vi "globalSetUp.vi"(8 "error in (no error)":errorcluster, 11 "Instrument Addon Error System Tests in":refnum<class "Instrument Addon Error System Tests.lvclass">) -> (0 "error out":errorcluster, 3 "Instrument Addon Error System Tests out":refnum<class "Instrument Addon Error System Tests.lvclass">)   [LabVIEW 2019, in "Instrument Addon Error System Tests.lvclass"]
uses:
  Instrument Addon Error System Tests.lvclass
  C:/Program Files (x86)/National Instruments/LabVIEW 2019/vi.lib/NI/VeriStand Custom Device Testing Tools/VeriStandTestCase/VeriStandTestCase.lvclass
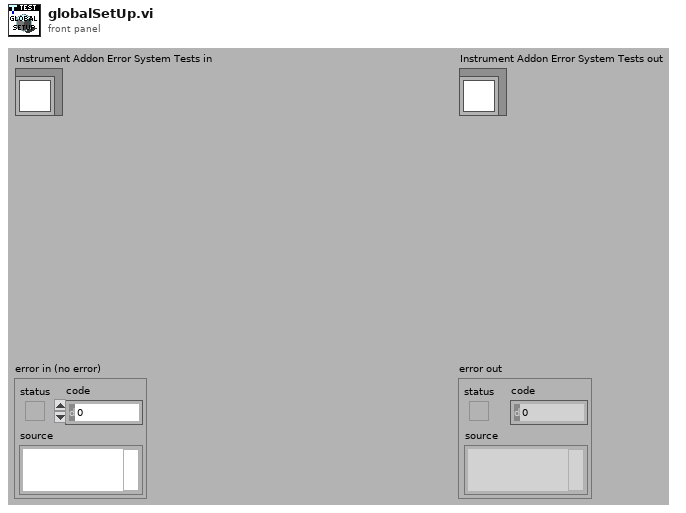
[diagram p1: front panel]
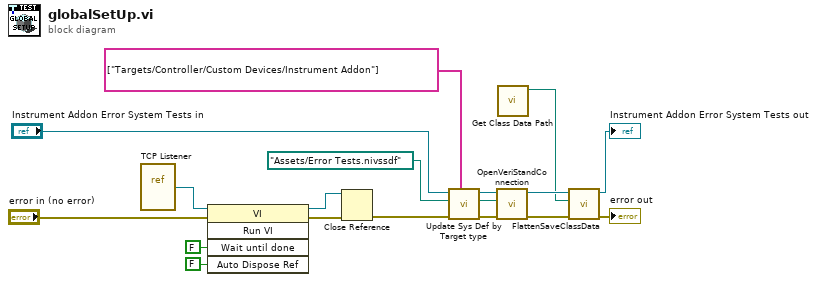
[diagram p0: block diagram]
diagram:
  n1 = vi-ref "TCP Listener.vi"() -> (w16:refnum<vi>)
  n2 = invoke class="VI" method="Run VI"(reference=w16, error in="error in (no error)", "Wait until done"=FALSE ("Wait Until Done"), "Auto Dispose Ref"=FALSE ("Auto Dispose Reference")) -> (reference out=w15:refnum<vi>, error out=w14:errorcluster)  [unwired: 1 in, 3 out]
  n3 = Close Reference(reference=w15, error in (no error)=w14) -> (error out=w5:errorcluster)
  n4 = call "Update Sys Def by Target type.vi"("nodepaths"=string[] ["Targets/Controller/Custom Devices/Instrument Addon"], "error in (no error)"=w5, "Sys Def relative path"=path "Assets/Error Tests.nivssdf" ("System Definition File"), "VeriStandTestCase in"="Instrument Addon Error System Tests in") -> ("error out"=w2:errorcluster, "Sys Def relative path out"=w3:path, "VeriStandTestCase out"=w6:refnum<class "Instrument Addon Error System Tests.lvclass">)  [unwired: 5 in]
  n5 = call-dynamic "OpenVeriStandConnection.vi"("error in (no error)"=w2, "System Definition File"=w3, "VeriStand Test Case in"=w6) -> ("error out"=w18:errorcluster, "VeriStand Test Case out"=w17:refnum<class "Instrument Addon Error System Tests.lvclass">)  [unwired: 6 in, 1 out]
  n6 = call "Get Class Data Path.vi"() -> ("Class Data File Path"=w8:path)  [unwired: 11 in]
  n7 = call-dynamic "FlattenSaveClassData.vi"("error in"=w18, "Class Data File Path"=w8, "VeriStandTestCase in"=w17) -> ("error out"=→"error out":errorcluster, "VeriStandTestCase out"=→"Instrument Addon Error System Tests out":refnum<class "Instrument Addon Error System Tests.lvclass">)  [unwired: 7 in]
